vi "Convert To Velocity Drive.vi"(8 "Abort Velocity Control":bool, 9 "Right Percent Output":dbl, 10 "Left Percent Output":dbl, 11 "Max Velocity Physically Allowed":dbl) -> (1 "Right Output":dbl, 2 "Left Output":dbl, 3 "Control Mode":T1 items=["PercentOutput"=0, "Position"=1, "Velocity"=2, "Current"=3, "Follower"=5, "MotionProfile"=6, "MotionMagic"=7, "MotionProfileArc"=10, "Disabled"=15])   [LabVIEW 2018]
uses:
  <vilib>/Rock Robotics/WPI/ThirdParty/Phoenix-LabVIEW/Motor Controller/Controls/CTRE_Phoenix_MotorControl_ControlMode.ctl
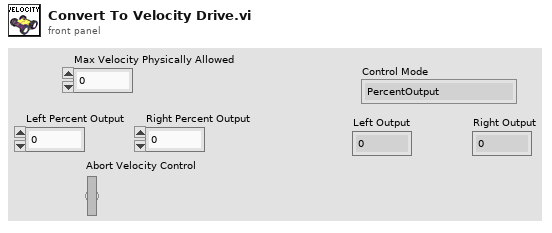
[diagram p1: front panel]
types:
  T1 = typedef "CTRE_Phoenix_MotorControl_ControlMode.ctl" = u16
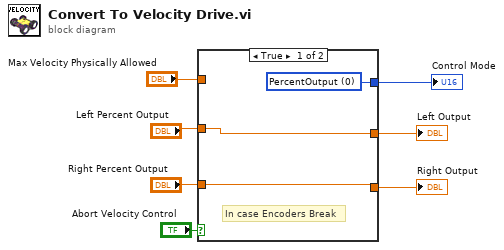
[diagram p0: block diagram]
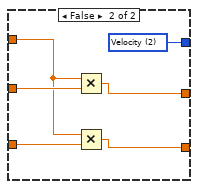
[diagram p2: hidden frame]
diagram:
  n1 = case shown="True" "Abort Velocity Control" {
    tunnel: "Right Percent Output" -> [w9 w16]
    tunnel: "Left Percent Output" -> [w10 w15]
    tunnel: "Max Velocity Physically Allowed" -> [_ w14]
    tunnel: [w10 w13] -> w3
    tunnel: [w9 w12] -> w2
    tunnel: [w8 w11] -> w1
    frame True {
      w8 = T1 0 items=["PercentOutput"=0, "Position"=1, "Velocity"=2, "Current"=3, "Follower"=5, "MotionProfile"=6, "MotionMagic"=7, "MotionProfileArc"=10, "Disabled"=15] ("Control Mode")
      # "In case Encoders Break"
    }
    frame False {
      w11 = T1 2 items=["PercentOutput"=0, "Position"=1, "Velocity"=2, "Current"=3, "Follower"=5, "MotionProfile"=6, "MotionMagic"=7, "MotionProfileArc"=10, "Disabled"=15] ("Control Mode")
      n2 = Multiply(x=w14, y=w15) -> (x*y=w13:dbl)
      n3 = Multiply(x=w14, y=w16) -> (x*y=w12:dbl)
    }
  }
  "Left Output" <- w3
  "Right Output" <- w2
  "Control Mode" <- w1
